vi "WiimoteEventHappenedCallback-IR.vi"(4 "Event args":refnum<vi>, 5 "Event Data":T1, 6 "Control Ref":refnum<k24>, 7 "Event Common Data":T2) -> ()   [LabVIEW 2010]
uses:
  C:/Users/×ñÞóôïò/Desktop/rtdsp_project14_4_11/3D_Experiment/libs/ola/WiimoteManaged(wml17)/WiimoteLib.dll
  WiimoteLib.dll
  wiimotestate.ctl
  wiimoteState(IR).ctl
panel:
  # "Accelerometers"
  # "Buttons"
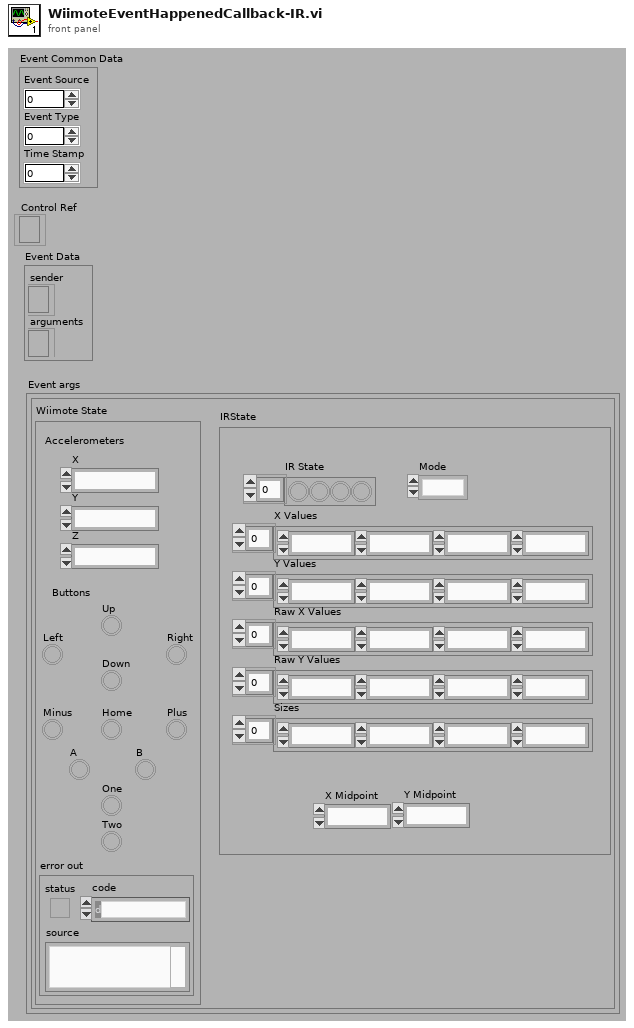
[diagram p1: front panel]
types:
  T1 = cluster{"sender":refnum<k24>, "arguments":refnum<k24>}
  T2 = cluster{"Event Source":i32, "Event Type":u32, "Time Stamp":u32}
  T3 = typedef "wiimotestate.ctl" = cluster{"X":sgl, "Y":sgl, "Z":sgl, "A":bool, "B":bool, "Down":bool, "Home":bool, "Left":bool, "Minus":bool, "One":bool, "Plus":bool, "Right":bool, "Two":bool, "Up":bool, "error out":errorcluster}
  T4 = typedef "wiimoteState(IR).ctl" = cluster{"Mode":u8, "IR State":bool[], "X Values":sgl[], "Y Values":sgl[], "Raw X Values":i32[], "Raw Y Values":i32[], "Sizes":i32[], "X Midpoint":sgl, "Y Midpoint":sgl}
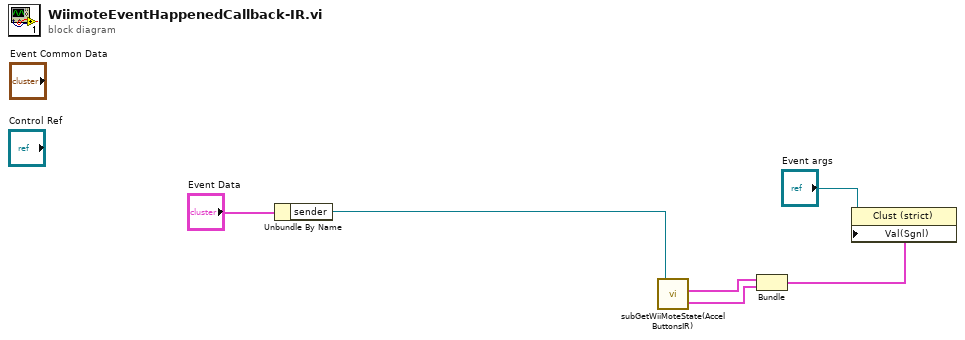
[diagram p0: block diagram]
diagram:
  n1 = Unbundle By Name("Event Data") -> ("sender"=w1:refnum<k24>)
  n2 = call "subGetWiiMoteState(AccelButtonsIR).vi"("Wiimote"=w1) -> ("Wiimote State"=w4:T3, "IRState"=w3:T4)  [unwired: 1 in, 2 out]
  n3 = Bundle("Wiimote State"=w4, "IRState"=w3) -> (w2:cluster{"Wiimote State":T3, "IRState":T4})  [unwired: 1 out]
  n4 = property class="Clust (strict)"(reference="Event args", "Val(Sgnl)"=w2) -> ()  [unwired: 1 in, 2 out]
